vi "InputModulus_Example.vi"() -> ()   [LabVIEW 2019]
uses:
  <vilib>/Rock Robotics/WPI/ThirdParty/JAS_Junk/TrajLib/Trajectory_Library.lvlib
panel:
  out "Input Moduls":dbl format="%14.3f"
  in  "Input":dbl(slide)=-0.015748031496062964 scale=-900.0..900.0
  out "Input Modulus":cluster{"Input":dbl, "Result":dbl}(graph)
  out "Raw Input":dbl=10.0 format="%14.3f"
  in  "Maximum_Input":dbl=180.0 format="%#_13g"
  in  "Minimum_Input":dbl=-180.0 format="%#_13g"
  # "Analog  - Input Modulus - Example"
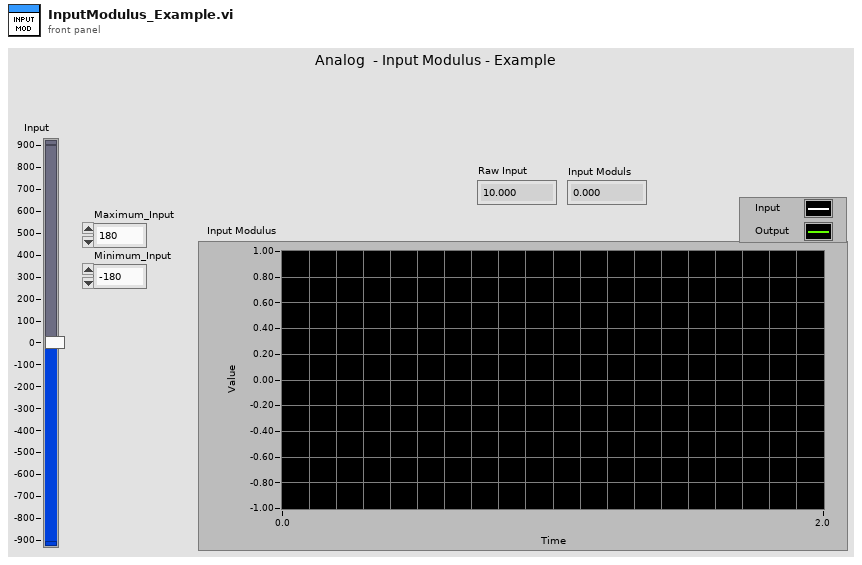
[diagram p1: front panel]
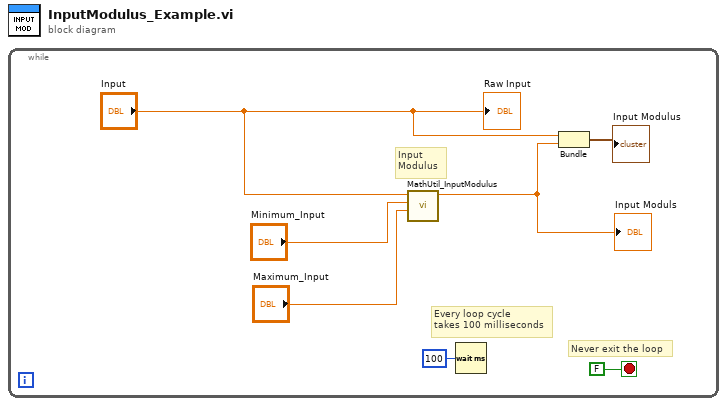
[diagram p0: block diagram]
diagram:
  n1 = while {
    stop <- FALSE stop-if-true
    # "Input\nModulus"
    # "Every loop cycle\ntakes 100 milliseconds"
    # "Never exit the loop"
    n2 = call <vilib>:"MathUtil_InputModulus.vi"("Maximum_Input"="Maximum_Input", "Minimum_Input"="Minimum_Input", "Input"="Input") -> ("modulus"=w1:dbl)  [unwired: 8 in]
    "Input Moduls" <- w1
    n3 = Wait (ms)(milliseconds to wait=u32 100) -> ()  [unwired: 1 out]
    n4 = Bundle("Input"="Input", "modulus"=w1) -> (→"Input Modulus":cluster{"Input":dbl, "modulus":dbl})  [unwired: 1 in]
    "Raw Input" <- "Input"
  }
